vi "IMAQ FPGA Pixel Bus to FIFO.vi"   [LabVIEW 2017, in "NI_VDM_FPGA_Basics.lvlib"]
doc: "Writes valid Pixel Data in the Pixel Bus cluster to the specified FIFO. If the FIFO is full, the Ready for Input terminal returns FALSE during that cycle."
uses:
  <vilib>/visionFPGA/NI_VDM_FPGA_Basics.lvlib
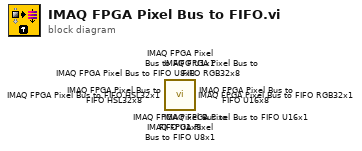
[diagram p0: block diagram]
diagram:
  n1 = call <vilib>:"IMAQ FPGA Pixel Bus to FIFO U1x8.vi"() -> ()  [unwired: 11 in, 1 out]
  n2 = call <vilib>:"IMAQ FPGA Pixel Bus to FIFO RGB32x8.vi"() -> ()  [unwired: 11 in, 1 out]
  n3 = call <vilib>:"IMAQ FPGA Pixel Bus to FIFO HSL32x8.vi"() -> ()  [unwired: 11 in, 1 out]
  n4 = call <vilib>:"IMAQ FPGA Pixel Bus to FIFO U16x8.vi"() -> ()  [unwired: 11 in, 1 out]
  n5 = call <vilib>:"IMAQ FPGA Pixel Bus to FIFO U8x8.vi"() -> ()  [unwired: 11 in, 1 out]
  n6 = call <vilib>:"IMAQ FPGA Pixel Bus to FIFO U1x1.vi"() -> ()  [unwired: 11 in, 1 out]
  n7 = call <vilib>:"IMAQ FPGA Pixel Bus to FIFO U16x1.vi"() -> ()  [unwired: 11 in, 1 out]
  n8 = call <vilib>:"IMAQ FPGA Pixel Bus to FIFO U8x1.vi"() -> ()  [unwired: 11 in, 1 out]
  n9 = call <vilib>:"IMAQ FPGA Pixel Bus to FIFO HSL32x1.vi"() -> ()  [unwired: 11 in, 1 out]
  n10 = call <vilib>:"IMAQ FPGA Pixel Bus to FIFO RGB32x1.vi"() -> ()  [unwired: 11 in, 1 out]
